vi "Depth and RGB Continuous Acquisition.vi"() -> ()   [LabVIEW 2011]
uses:
  <vilib>/LabVIEW Hacker/LVH-Interface-for-Kinect/LVH-Interface-for-Kinect.lvlib
panel:
  out "Kinect Depth Image":T1(plugin-control)
  out "Kinect RGB Image":T1(plugin-control)
  out "Frame Number":i32
  in  "Stop Button":bool
  # "This example continuously acquires the depth and RGB images from the Kinect ."
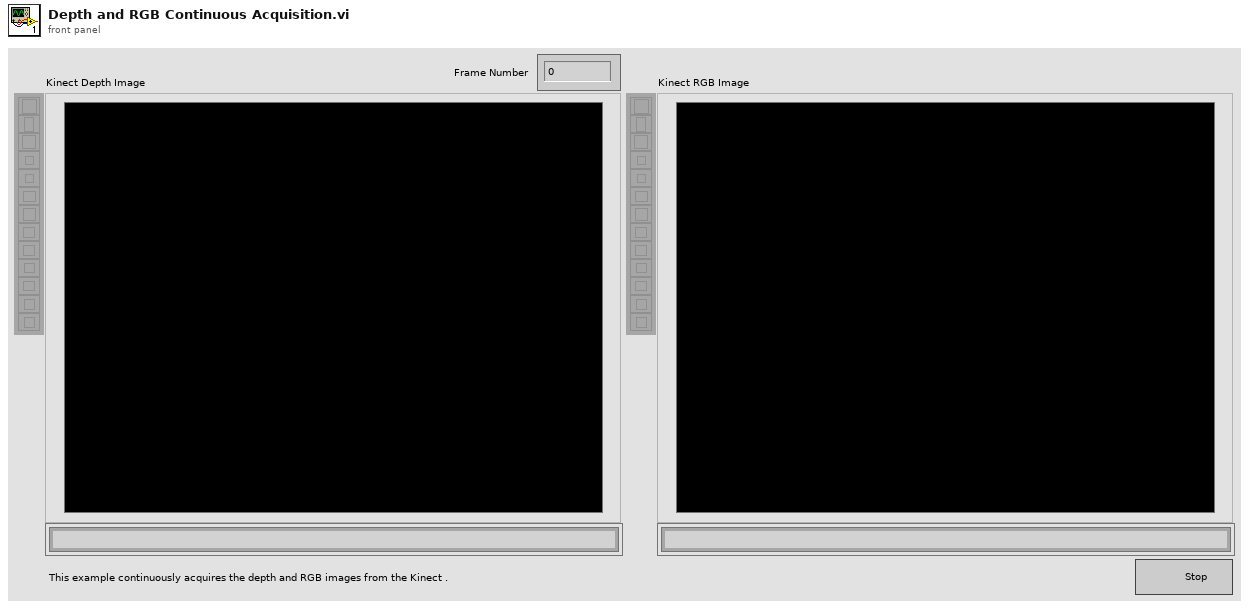
[diagram p1: front panel]
types:
  T1 = typedef "IMAQ Image.ctl" = refnum<image>
  T2 = typedef "Image Type" = u32
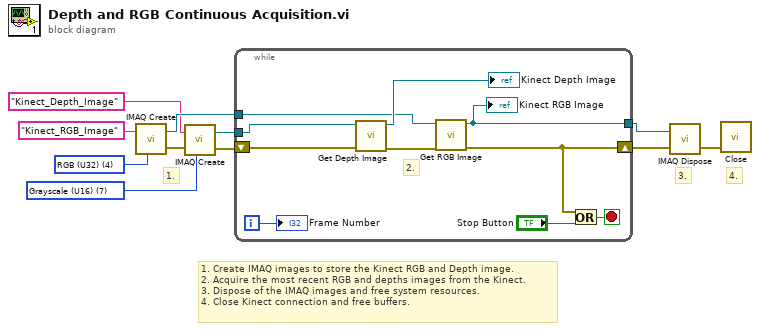
[diagram p0: block diagram]
diagram:
  w1 = T2 7 items=["Grayscale (U8)", "Grayscale (I16)", "Grayscale (SGL)", "Complex (CSG)", "RGB (U32)", "HSL (U32)", "RGB (U64)", "Grayscale (U16)"] ("Image Type")
  w10 = T2 4 items=["Grayscale (U8)", "Grayscale (I16)", "Grayscale (SGL)", "Complex (CSG)", "RGB (U32)", "HSL (U32)", "RGB (U64)", "Grayscale (U16)"] ("Image Type")
  # "4."
  # "1. Create IMAQ images to store the Kinect RGB and Depth image.\n2. Acquire the most recent RGB and depths images from the Kinect.\n3. Dispose of the IMAQ images and free system resources.\n4. Close Kinect connection and free buffers."
  # "3."
  # "1."
  n1 = call "IMAQ Create"("Image Name"="Kinect_RGB_Image", "Image Type"=w10) -> ("New Image"=w4:T1, "error out"=w7:errorcluster)  [unwired: 3 in]
  n2 = call "IMAQ Create"("Image Name"="Kinect_Depth_Image", "Image Type"=w1, "error in (no error)"=w7) -> ("New Image"=w5:T1, "error out"=w6:errorcluster)  [unwired: 2 in]
  n3 = while {
    tunnel: [w13] -> w11
    shift-right: [w18] -> w9
    shift-left: w6 -> [w17]
    tunnel: w5 -> [w16]
    tunnel: w4 -> [w12]
    i -> [w21]
    stop <- w19 stop-if-true
    # "2."
    n4 = call <vilib>:"Get Depth Image.vi"("Error In"=w17, "Image"=w16) -> ("Error Out"=w14:errorcluster, "Image Out"=→"Kinect Depth Image":T1)  [unwired: 7 in, 1 out]
    n5 = call <vilib>:"Get RGB Image.vi"("Error In"=w14, "Image"=w12) -> ("Error Out"=w18:errorcluster, "Image Out"=w13:T1)  [unwired: 7 in, 1 out]
    "Kinect RGB Image" <- w13
    n6 = Or(x=w18, y="Stop Button") -> (x .or. y?=w19:bool)
    "Frame Number" <- w21
  }
  n7 = call "IMAQ Dispose"("Image"=w11, "error in (no error)"=w9) -> ("error out"=w8:errorcluster)  [unwired: 4 in]
  n8 = call <vilib>:"Close.vi"("Error In"=w8) -> ()  [unwired: 10 in, 1 out]
